vi "test 单通道.vi"() -> ()   [LabVIEW 2023]
uses:
  <vilib>/Utility/file.llb/Write Delimited Spreadsheet (DBL).vi
  vmmsolib/vmmsolib.lvlib
panel:
  out "Capture is OK? 2":bool=TRUE
  out "function return":i32
  in  "探头1":dbl(ring)=10.0 items=["X1"=1.0, "X10"=10.0]
  out "混合信号图":dbl[](graph)
  out "x = y?":bool=TRUE
  out "Device is OK?":bool=TRUE
  in  "保存\n按钮":bool
  in  "空白按钮":bool
  out "ReadVoltageData Return":u32=10240
  in  "储存深度 （k Points）":i32=10
  in  "采集开关":bool=TRUE
  out "数值":i32=744
  in  "Trigger Sense （div）":dbl=0.1
  in  "Pre-Trigger Percent":i32=50
  in  "Trigger Level （mv）":i32=100
  in  "触发类型选择":u32(ring)=1 items=["Not Trigger"=0, "RIsing Edge"=1, "Falling Edge"=2, "Edge"=4, "Positive Pulse width(>)"=8, "Positive Pulse width(<)"=16, "Positive Pulse width(<>)"=32, "Negativea Pulse width(>)"=64, "Negativea Pulse width(<)"=128, "Negativea Pulse width(<>)"=256]
  in  "触发模式选择":u32(ring)=1 items=["AUTO", "LIANXU"]
  in  "触发通道选择":u32(ring) items=["Channel1", "Channel2"]
  in  "触发开关":bool
  in  "采样频率设置":i32=9
  out "Support Samples （MHz）":dbl[](array[numeric])=[0.001, 0.002, 0.005, 0.01, 0.02, 0.049999999999999996, 0.09999999999999999, 0.19999999999999998, 0.5, 1.0, 2.0, 5.0, 10.0, 20.0, 50.0, 100.0, 200.0, 0.0, 0.0, 0.0, 0.0, 0.0, 0.0, 0.0, 0.0, 0.0, 0.0, 0.0, 0.0, 0.0, 0.0, 0.0, 0.0, 0.0, 0.0, 0.0, 0.0, 0.0, 0.0, 0.0, 0.0, 0.0, 0.0, 0.0, 0.0, 0.0, 0.0, 0.0, 0.0, 0.0, 0.0, 0.0, 0.0, 0.0, 0.0, 0.0, 0.0, 0.0, 0.0, 0.0]
  # "物理设备状态"
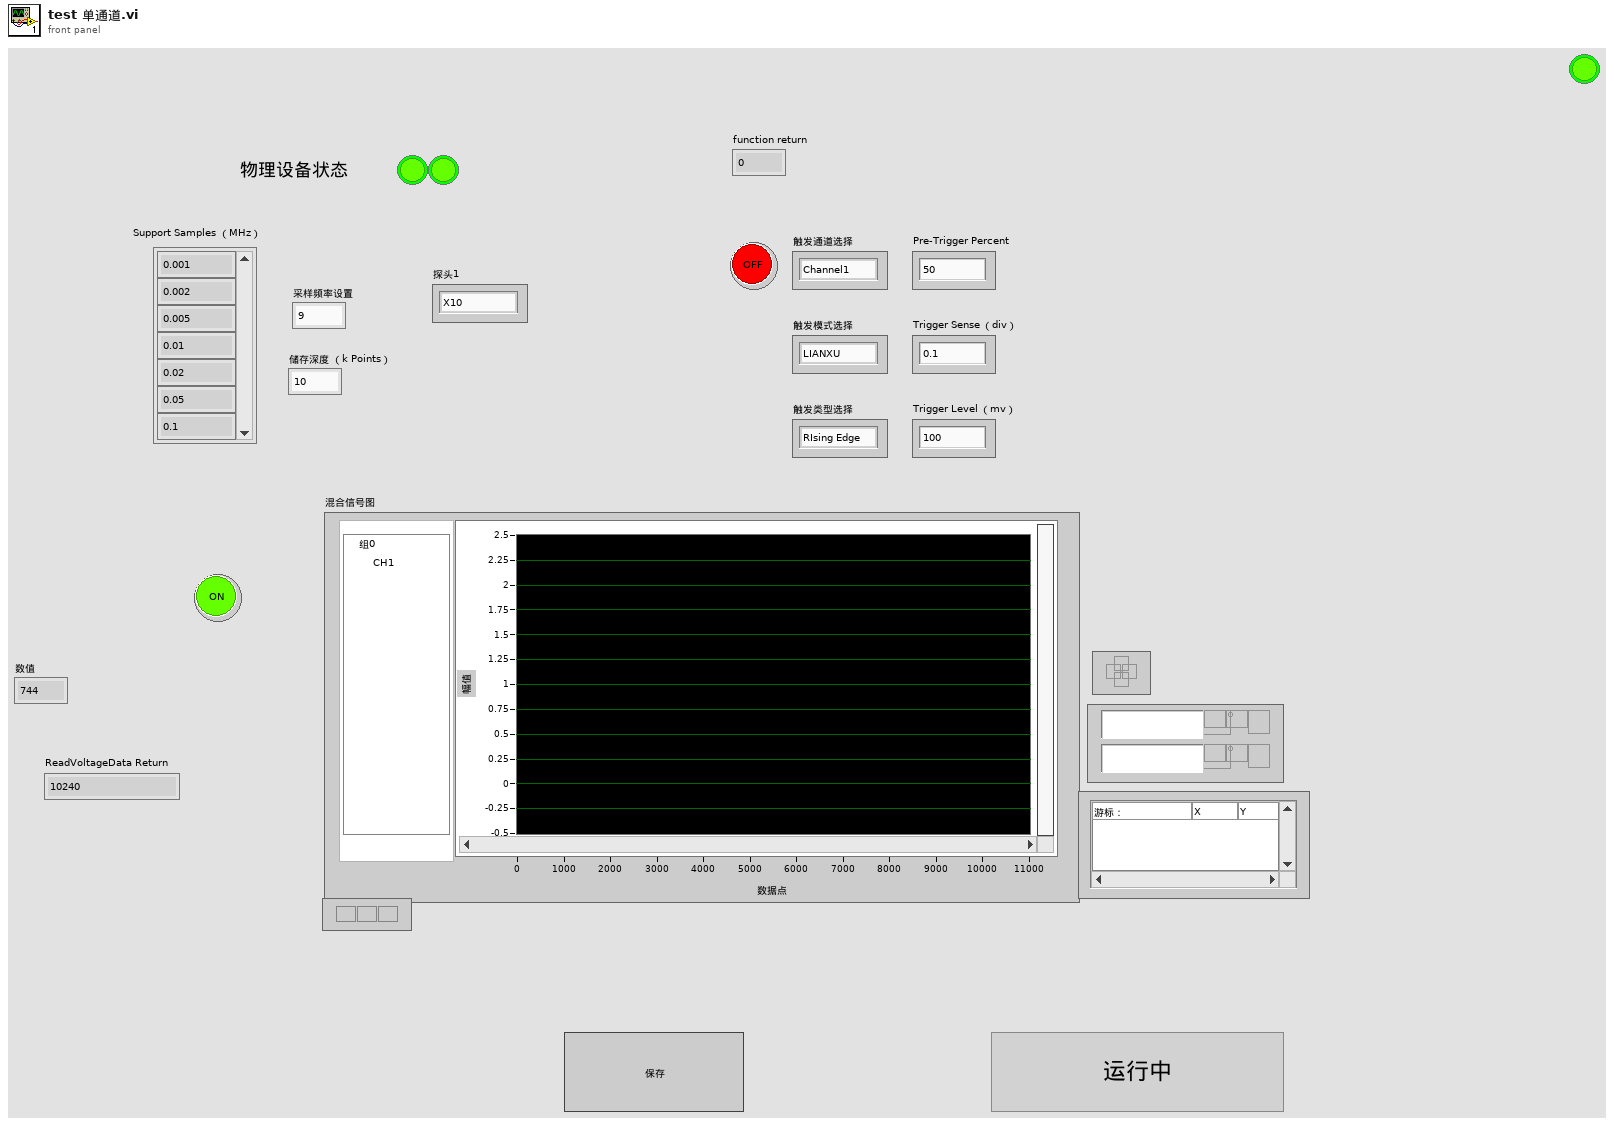
[diagram p1: front panel]
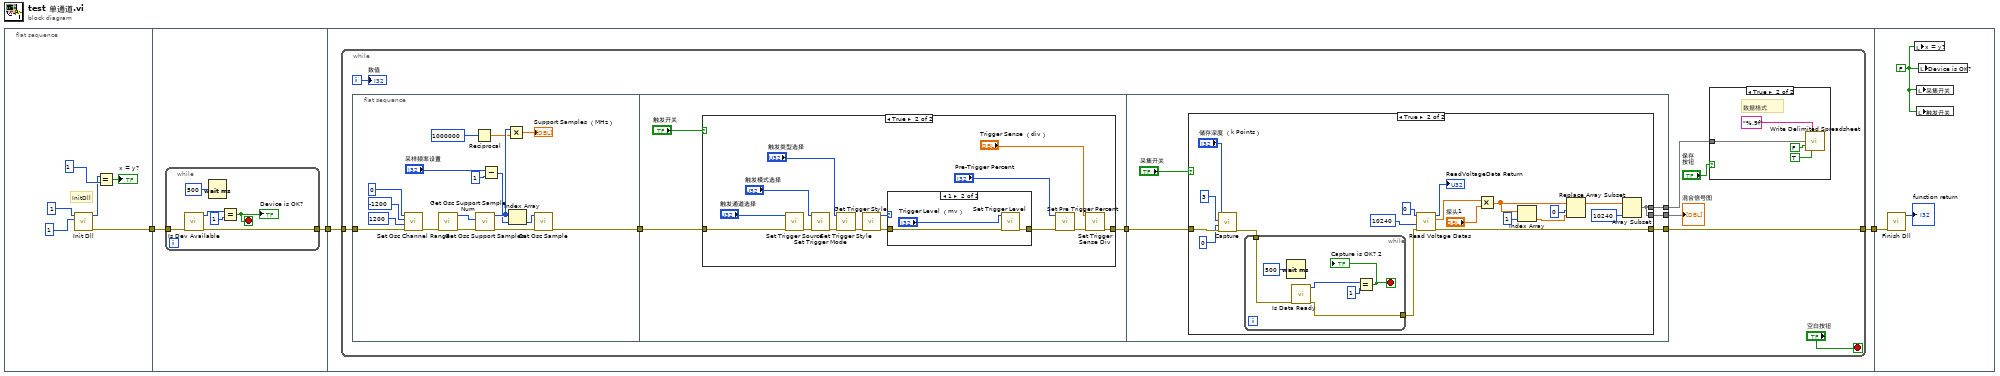
[diagram p0: block diagram]
diagram:
  n1 = flat-sequence {
    tunnel: [w6] -> w3
    tunnel: w3 -> [w11]
    tunnel: [w10] -> w2
    tunnel: w2 -> [w19]
    tunnel: [w18] -> w1
    tunnel: w1 -> [w100]
    frame #0 {
      # "InitDll"
      n2 = call "Init Dll.vi"("en_hard_watchdog"=1 ("y"), "en_log"=1 ("y")) -> ("error out"=w6:errorcluster, "function return"=w7:i32)  [unwired: 8 in]
      n3 = Equal?(x=w7, y=1) -> (x = y?=→"x = y?":bool)
    }
    frame #1 {
      n4 = while {
        tunnel: w11 -> [w13]
        tunnel: [w12] -> w10
        stop <- w15 stop-if-true
        n5 = call "Is Dev Available.vi"("error in (no error)"=w13) -> ("error out"=w12:errorcluster, "function return"=w14:i32)  [unwired: 9 in]
        n6 = Wait (ms)(milliseconds to wait=u32 500 ("等待时间（毫秒）")) -> ()  [unwired: 1 out]
        n7 = Equal?(x=w14, y=1) -> (x = y?=w15:bool)
        "Device is OK?" <- w15
      }
    }
    frame #2 {
      n8 = while {
        tunnel: w19 -> [w20]
        tunnel: [w23] -> w18
        i -> [w28]
        stop <- "空白按钮" stop-if-true
        n9 = flat-sequence {
          tunnel: [w34] -> w25
          tunnel: w20 -> [w33]
          tunnel: w25 -> [w47]
          tunnel: [w46] -> w24
          tunnel: w24 -> [w70]
          tunnel: [w69] -> w23
          tunnel: [w67] -> w22
          tunnel: [w66] -> w21
          frame #0 {
            n10 = call "Set Osc Channel Range.vi"("error in (no error)"=w33, "maxmv"=1200, "minmv"=-1200, "channel"=0) -> ("error out"=w32:errorcluster)  [unwired: 6 in, 1 out]
            n11 = call "Get Osc Support Sample Num.vi"("error in (no error)"=w32) -> ("error out"=w44:errorcluster, "function return"=w43:i32)  [unwired: 9 in]
            n12 = Reciprocal(x=1000000) -> (1/x=w42:dbl)
            n13 = call "Get Osc Support Samples.vi"("error in (no error)"=w44, "maxnum"=w43) -> ("error out"=w40:errorcluster, "sample out"=w45:u32[])  [unwired: 7 in, 1 out]
            n14 = Subtract(x="采样频率设置", y=1) -> (x-y=w39:i32)
            n15 = Multiply(x=w45, y=w42) -> (x*y=→"Support Samples （MHz）":dbl[])
            n16 = Index Array(array=w45, index=w39) -> (element=w38:u32)
            n17 = call "Set Osc Sample.vi"("error in (no error)"=w40, "sample"=w38) -> ("error out"=w34:errorcluster)  [unwired: 8 in, 1 out]
          }
          frame #1 {
            n18 = case shown="True" "触发开关" {
              tunnel: w47 -> [_ w62]
              tunnel: [_ w49] -> w46
              frame False {
              }
              frame True {
                n19 = call "Set Trigger Source.vi"("error in (no error)"=w62, "source"="触发通道选择") -> ("error out"=w60:errorcluster)  [unwired: 9 in]
                n20 = call "Set Trigger Mode.vi"("error in (no error)"=w60, "mode"="触发模式选择") -> ("error out"=w58:errorcluster)  [unwired: 9 in]
                n21 = call "Set Trigger Style.vi"("error in (no error)"=w58, "style"="触发类型选择") -> ("error out"=w56:errorcluster)  [unwired: 9 in]
                n22 = call "Get Trigger Style.vi"("error in (no error)"=w56) -> ("error out"=w54:errorcluster, "function return"=w55:u32)  [unwired: 9 in]
                n23 = case shown="1" w55 {
                  tunnel: w54 -> [_ w65]
                  tunnel: [_ w63] -> w50
                  frame 0, Default {
                  }
                  frame 1 {
                    n24 = call "Set Trigger Level.vi"("error in (no error)"=w65, "level"="Trigger Level （mv）") -> ("error out"=w63:errorcluster)  [unwired: 9 in]
                  }
                }
                n25 = call "Set Pre Trigger Percent.vi"("error in (no error)"=w50, "front"="Pre-Trigger Percent") -> ("error out"=w52:errorcluster)  [unwired: 9 in]
                n26 = call "Set Trigger Sense Div.vi"("error in (no error)"=w52, "sense"="Trigger Sense （div）") -> ("error out"=w49:errorcluster)  [unwired: 9 in]
              }
            }
          }
          frame #2 {
            n27 = case shown="True" "采集开关" {
              tunnel: w70 -> [_ w89]
              tunnel: [_ w88] -> w69
              tunnel: [_ w81] -> w67
              tunnel: [_ w81] -> w66
              frame False {
              }
              frame True {
                n28 = call "Capture.vi"("error in (no error)"=w89, "force_length"=u16 0 ("capture_channel"), "capture_channel"=u16 3, "length"="储存深度 （k Points）") -> ("error out"=w72:errorcluster)  [unwired: 6 in, 1 out]
                n29 = while {
                  tunnel: w72 -> [w92]
                  tunnel: [w91] -> w71
                  stop <- w93 stop-if-true
                  n30 = Wait (ms)(milliseconds to wait=u32 500 ("等待时间（毫秒）")) -> ()  [unwired: 1 out]
                  n31 = call "Is Data Ready.vi"("error in (no error)"=w92) -> ("error out"=w91:errorcluster, "function return"=w90:i32)  [unwired: 9 in]
                  n32 = Equal?(x=w90, y=1) -> (x = y?=w93:bool)
                  "Capture is OK? 2" <- w93
                }
                n33 = call "Read Voltage Datas.vi"("error in (no error)"=w71, "length"=u32 10240, "channel"=i8 0) -> ("error out"=w88:errorcluster, "buffer out"=w78:dbl[], "function return"=→"ReadVoltageData Return":u32)  [unwired: 6 in]
                n34 = Multiply(x=w78, y="探头1") -> (x*y=w84:dbl[])
                n35 = Index Array(array=w84, index=1 ("索引")) -> (element=w83:dbl)
                n36 = Replace Array Subset(array=w84, new element=w83, index=0 ("索引")) -> (w82:dbl[])
                n37 = Array Subset(array=w82, length=10240 ("长度")) -> (w81:dbl[])  [unwired: 1 in]
              }
            }
          }
        }
        n38 = case shown="True" "保存\n按钮" {
          tunnel: w21 -> [_ w96]
          frame False {
          }
          frame True {
            # "数据格式"
            n39 = call-poly <vilib>:"Write Delimited Spreadsheet.vi"("format (%.3f)"="%.9f", "1D data"=w96, "append to file? (new file:F)"=FALSE, "transpose? (no:F)"=TRUE) -> ()  [unwired: 10 in, 2 out]
          }
        }
        "数值" <- w28
        "混合信号图" <- w22
      }
    }
    frame #3 {
      w102 = FALSE
      n40 = call "Finish Dll.vi"("error in (no error)"=w100) -> ("function return"=→"function return":i32)  [unwired: 9 in, 1 out]
      n41 = local write "x = y?"(w102) -> ()
      n42 = local write "采集开关"(w102) -> ()
      n43 = local write "触发开关"(w102) -> ()
      n44 = local write "Device is OK?"(w102) -> ()
    }
  }
